vi "Apply Source Settings.vi"(5 "Include ?":bool=TRUE, 7 "Source Index":i32, 8 "error in (no error)":errorcluster, 10 "Source Type":string, 11 "BuildSpec in":refnum<vi>) -> (0 "error out":errorcluster, 3 "BuildSpec out":refnum<vi>)   [LabVIEW 2019, in "Project Sync Tools.lvclass"]
uses:
  Project Sync Tools.lvclass
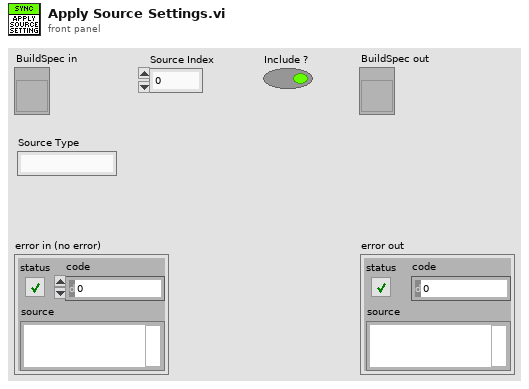
[diagram p1: front panel]
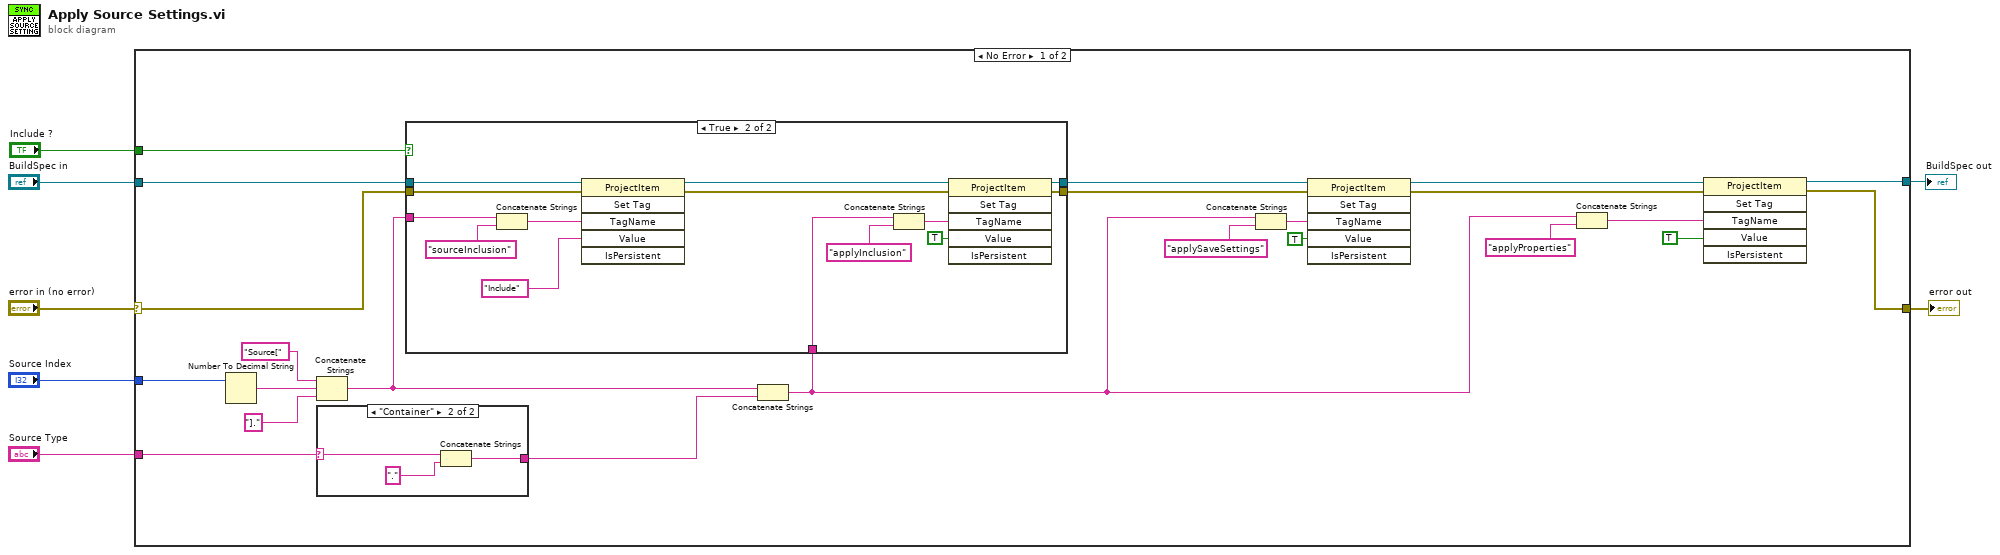
[diagram p0: block diagram]
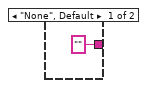
[diagram p3: hidden frame]
diagram:
  n1 = case shown="No Error" "error in (no error)" {
    selector: "error in (no error)" -> [w9 w51]
    tunnel: "BuildSpec in" -> [w30 w52]
    tunnel: [w29 w51] -> w6
    tunnel: [w28 w52] -> w5
    tunnel: "Source Index" -> [w20 _]
    tunnel: "Source Type" -> [w18 _]
    tunnel: "Include ?" -> [w8 _]
    frame No Error {
      n2 = Number To Decimal String(number=w20) -> (decimal integer string=w22:string)  [unwired: 1 in]
      n3 = Concatenate Strings("Source[" ("string"), w22, "].") -> (w19:string)
      n4 = case shown="\"Container\"" w18 {
        selector: w18 -> [_ w50]
        tunnel: ["" w48] -> w17
        frame "None", Default {
        }
        frame "Container" {
          n5 = Concatenate Strings(w50, ".") -> (w48:string)
        }
      }
      n6 = Concatenate Strings(w19, w17) -> (w13:string)
      n7 = case shown="True" w8 {
        tunnel: w30 -> [w32 w44]
        tunnel: [w31 w43] -> w27
        tunnel: [w32 w42] -> w24
        tunnel: w19 -> [_ w38]
        tunnel: w13 -> [_ w35]
        tunnel: w9 -> [w31 w33]
        frame False {
        }
        frame True {
          n8 = Concatenate Strings(w38, "sourceInclusion") -> (w39:string)
          n9 = invoke class="ProjectItem" method="Set Tag"(reference=w44, error in=w33, "TagName"=w39, "Value"="Include") -> (reference out=w45:refnum<vi>, error out=w46:errorcluster)  [unwired: 2 in, 4 out]
          n10 = Concatenate Strings(w35, "applyInclusion") -> (w36:string)
          n11 = invoke class="ProjectItem" method="Set Tag"(reference=w45, error in=w46, "TagName"=w36, "Value"=TRUE) -> (reference out=w42:refnum<vi>, error out=w43:errorcluster)  [unwired: 2 in, 4 out]
        }
      }
      n12 = Concatenate Strings(w13, "applySaveSettings") -> (w15:string)
      n13 = invoke class="ProjectItem" method="Set Tag"(reference=w24, error in=w27, "TagName"=w15, "Value"=TRUE) -> (reference out=w25:refnum<vi>, error out=w26:errorcluster)  [unwired: 2 in, 4 out]
      n14 = Concatenate Strings(w13, "applyProperties") -> (w12:string)
      n15 = invoke class="ProjectItem" method="Set Tag"(reference=w25, error in=w26, "TagName"=w12, "Value"=TRUE) -> (reference out=w28:refnum<vi>, error out=w29:errorcluster)  [unwired: 2 in, 4 out]
    }
    frame Error {
    }
  }
  "error out" <- w6
  "BuildSpec out" <- w5
